vi "Toolbar Tree.vi"   [LabVIEW 2011, in "Toolbar Control.lvclass"]
doc: "-------------\nDeveloped by Brian Hoover (hooovahh)"
uses:
  Toolbar Control.lvclass
  Add Icon From Path.vi
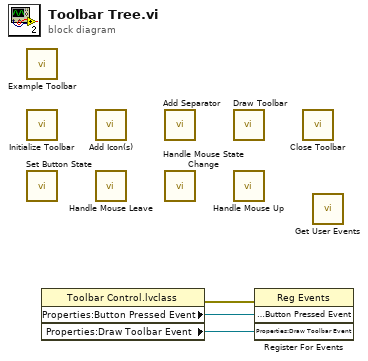
[diagram p0: block diagram]
diagram:
  n1 = call "Example Toolbar.vi"() -> ()  [unwired: 12 in]
  n2 = call "Initialize Toolbar.vi"() -> ()  [unwired: 10 in, 2 out]
  n3 = call "Set Button State.vi"() -> ()  [unwired: 9 in, 3 out]
  n4 = property class="Toolbar Control.lvclass"() -> (error out=w1:errorcluster, "Properties:Button Pressed Event"=w2:refnum<user-event>, "Properties:Draw Toolbar Event"=w3:refnum<user-event>)  [unwired: 2 in, 1 out]
  n5 = call-poly "Add Icon(s).vi"() -> ()  [unwired: 10 in, 2 out]
  n6 = call "Handle Mouse Leave.vi"() -> ()  [unwired: 9 in, 3 out]
  n7 = call "Add Separator.vi"() -> ()  [unwired: 10 in, 2 out]
  n8 = call "Handle Mouse State Change.vi"() -> ()  [unwired: 8 in, 4 out]
  n9 = call "Draw Toolbar.vi"() -> ()  [unwired: 9 in, 3 out]
  n10 = call "Handle Mouse Up.vi"() -> ()  [unwired: 7 in, 5 out]
  n11 = register-events(error in=w1, w2, w3) -> ()  [unwired: 1 in, 2 out]
  n12 = call "Close Toolbar.vi"() -> ()  [unwired: 11 in, 1 out]
  n13 = call "Get User Events.vi"() -> ()  [unwired: 12 in]
